vi "Convert Seconds to String.vi"(11 "Time In":dbl) -> (3 "String Out":string)   [LabVIEW 2019]
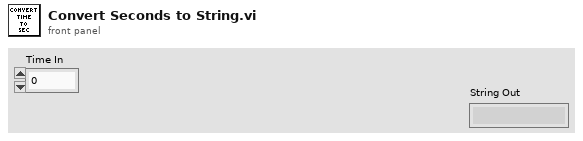
[diagram p1: front panel]
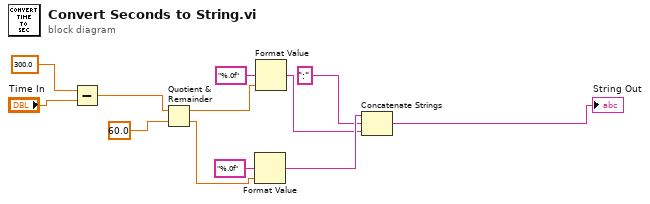
[diagram p0: block diagram]
diagram:
  n1 = Subtract(x=300.0, y="Time In") -> (x-y=w9:dbl)
  n2 = Quotient & Remainder(x=w9, y=60.0) -> (x-y*floor(x/y)=w5:dbl, floor(x/y)=w7:dbl)
  n3 = Format Value(format string="%.0f", value (0)=w7) -> (output string=w4:string)  [unwired: 1 in]
  n4 = Format Value(format string="%.0f", value (0)=w5) -> (output string=w2:string)  [unwired: 1 in]
  n5 = Concatenate Strings(w4, ":" ("string"), w2) -> (→"String Out":string)
